vi "Global Thermistor Coefficient Array.vi"() -> ()   [LabVIEW 2019]
panel:
  in  "Fit Coefficients":dbl[][](array[numeric])
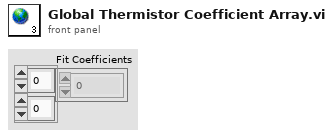
[diagram p1: front panel]
diagram:
